vi "Generate Pulse.vi"(8 "error in (no error)":errorcluster, 10 "Noise":dbl, 11 "EmulatorActor in":refnum<class "EmulatorActor.lvclass">) -> (0 "error out":errorcluster, 3 "EmulatorActor out":refnum<class "EmulatorActor.lvclass">)   [LabVIEW 2019, in "EmulatorActor.lvlib" / "EmulatorActor.lvclass"]
uses:
  EmulatorActor.lvclass
  EmulatorActor.lvclass/EmulatorActor.ctl
  DigitiserActor/DigitiserActor Messages/Process Data Msg/Process Data Msg.lvclass/Process Data Msg.ctl
  <vilib>/ActorFramework/Message Enqueuer/Message Enqueuer.lvclass/Message Enqueuer.ctl
  <vilib>/ActorFramework/Message Enqueuer/Enqueue.vi
  DigitiserActor/DigitiserActor Messages/Process Data Msg/Process Data Msg.lvclass
  C:/Program Files (x86)/National Instruments/LabVIEW 2019/vi.lib/ActorFramework/Message/Message.lvclass
  <vilib>/ActorFramework/Message Priority Queue/Priority Enqueue.vi
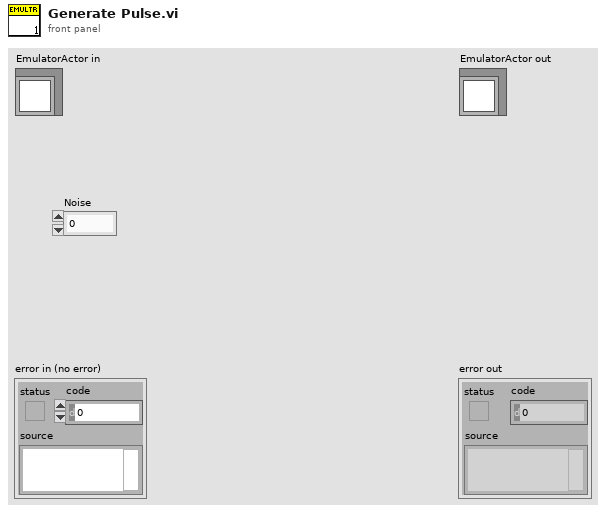
[diagram p1: front panel]
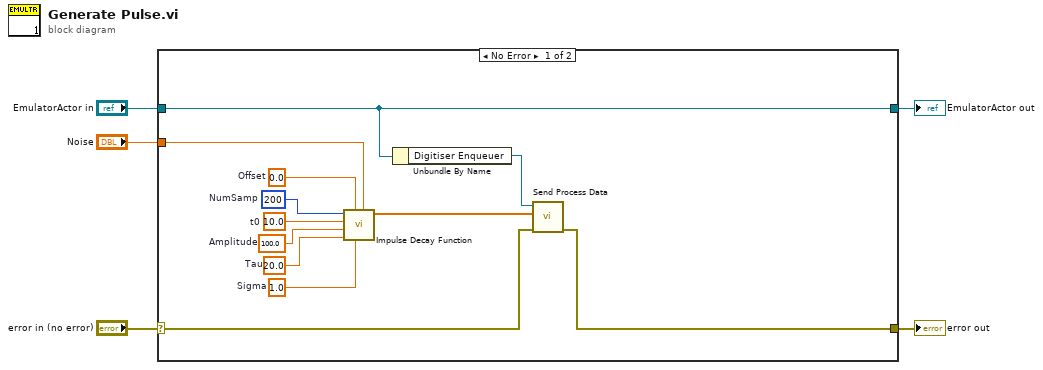
[diagram p0: block diagram]
diagram:
  n1 = case shown="No Error" "error in (no error)" {
    selector: "error in (no error)" -> [w8 w19]
    tunnel: [w7 w19] -> w4
    tunnel: [w6 w18] -> w2
    tunnel: "EmulatorActor in" -> [w6 w18]
    tunnel: "Noise" -> [w11 _]
    frame No Error {
      w12 = 0.0  # Offset
      w13 = u16 200  # NumSamp
      w14 = 10.0  # t0
      w15 = 100.0  # Amplitude
      w16 = 20.0  # Tau
      w17 = 1.0  # Sigma
      n2 = call "Impulse Decay Function.vi"("Noise"=w11, "Sigma"=w17, "Offset"=w12, "Tau"=w16, "Amplitude"=w15, "t0"=w14, "NumSamp"=w13) -> ("Array out"=w9:dbl[])  [unwired: 4 in]
      n3 = Unbundle By Name(w6) -> ("Digitiser Enqueuer"=w10:refnum<class "Message Enqueuer.lvclass">)
      n4 = call "Send Process Data.vi"("error in (no error)"=w8, "Raw Pulse In"=w9, "Message Enqueuer"=w10) -> ("error out"=w7:errorcluster)  [unwired: 7 in, 1 out]
    }
    frame Error {
    }
  }
  "error out" <- w4
  "EmulatorActor out" <- w2
